vi "ReadObjectLayout.vi"(7 "properties to ignore":variant, 8 "error in (no error)":errorcluster, 10 "GObj Refnum":refnum<vi>, 11 "String Control Layout in":refnum<class "String Control Layout.lvclass">) -> (0 "error out":errorcluster, 3 "String Control Layout out":refnum<class "String Control Layout.lvclass">)   [LabVIEW 2010, in "NI_SE_Front Panel Layout.lvlib" / "String Control Layout.lvclass"]
doc: "Read layout information from the GObj Refnum."
uses:
  String Control Layout.lvclass
  Control Layout/Control Layout.lvclass
  String Control Layout.lvclass/String Control Layout.ctl
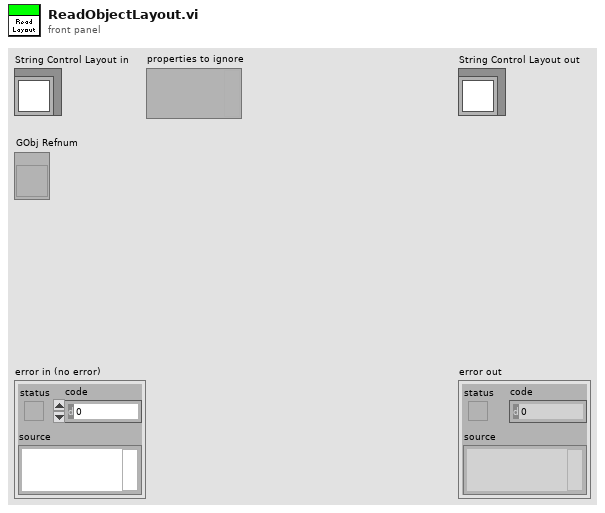
[diagram p1: front panel]
types:
  T1 = typedef "LVFontTypeDef.ctl" = cluster{"Font Name":string, "Size":u16, "Bold":bool, "Italic":bool, "Underline":bool, "Strikeout":bool, "Color":u32}
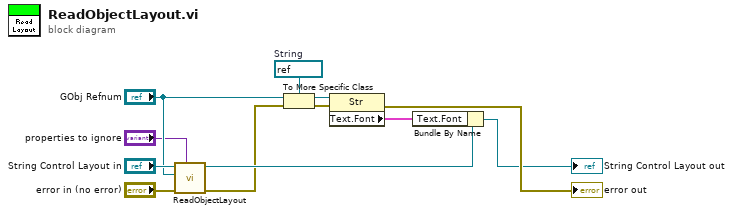
[diagram p0: block diagram]
diagram:
  w4 = refnum<vi> refnum  # String
  n1 = call-parent "ReadObjectLayout.vi"("properties to ignore"="properties to ignore", "error in (no error)"="error in (no error)", "GObj Refnum"="GObj Refnum", "Control Layout in"="String Control Layout in") -> ("error out"=w9:errorcluster, "Control Layout out"=w10:refnum<class "String Control Layout.lvclass">)  [unwired: 6 in]
  n2 = To More Specific Class(target class=w4, reference="GObj Refnum", error in=w9) -> (specific class reference=w3:refnum<vi>, error out=w2:errorcluster)
  n3 = property class="Str"(reference=w3, error in=w2) -> (error out=→"error out":errorcluster, "Text.Font"=w1:T1)  [unwired: 1 out]
  n4 = Bundle By Name(cluster=w10, "Text.Font"=w1) -> (→"String Control Layout out":refnum<class "String Control Layout.lvclass">)
